vi "Manual Shooter Mode.vi"(9 "Shoooooot RPM":dbl, 10 "manUEL Control Cluster":T1) -> (1 "da hoood":bool, 2 "Hopper Speed":dbl, 3 "Shot RPM":dbl)   [LabVIEW 2016]
uses:
  Common Code/Manual Shoot Cluster.ctl
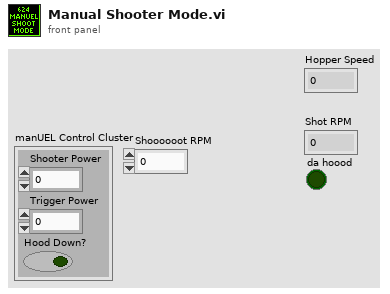
[diagram p1: front panel]
types:
  T1 = typedef "Manual Shoot Cluster.ctl" = cluster{"Shooter Power":dbl, "Hood Down?":bool, "Trigger Power":dbl}
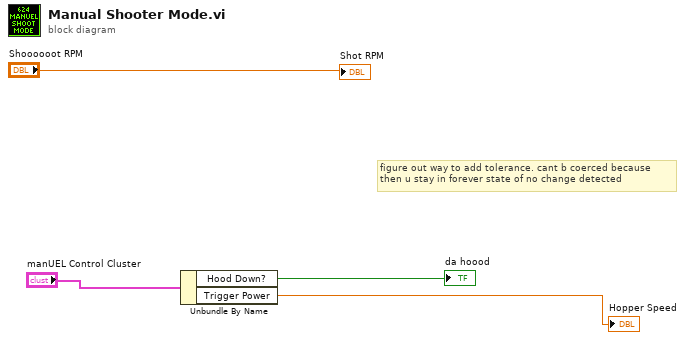
[diagram p0: block diagram]
diagram:
  # "figure out way to add tolerance. cant b coerced because\nthen u stay in forever state of no change detected"
  n1 = Unbundle By Name("manUEL Control Cluster") -> ("Hood Down?"=→"da hoood":bool, "Trigger Power"=→"Hopper Speed":dbl)
  "Shot RPM" <- "Shoooooot RPM"
